vi "Power Values (Single Line).vi"(0 "phase voltage spectra":T2(array[cluster]), 5 "current spectra":T2(array[cluster]), 9 "system info in":refnum<class "EP System Info.lvclass">, 11 "error in (no error)":errorcluster) -> (4 "power values":T4, 6 "total power values":T3, 10 "system info out":refnum<class "EP System Info.lvclass">, 15 "error out":errorcluster)   [LabVIEW 2013, in "NI_EP_Power Quality.lvlib"]
doc: "Calculates the power values from the voltage and current spectra."
uses:
  <vilib>/addons/Electrical Power/PQ/NI_EP_Power Quality.lvlib
  <vilib>/addons/Electrical Power/PQ/Common/Classes/System Info/EP System Info.lvclass
  <vilib>/addons/Electrical Power/PQ/Common/Controls/ep_AI Data Channel.ctl
  <vilib>/addons/Electrical Power/Basic/NI_EP_Basic.lvlib
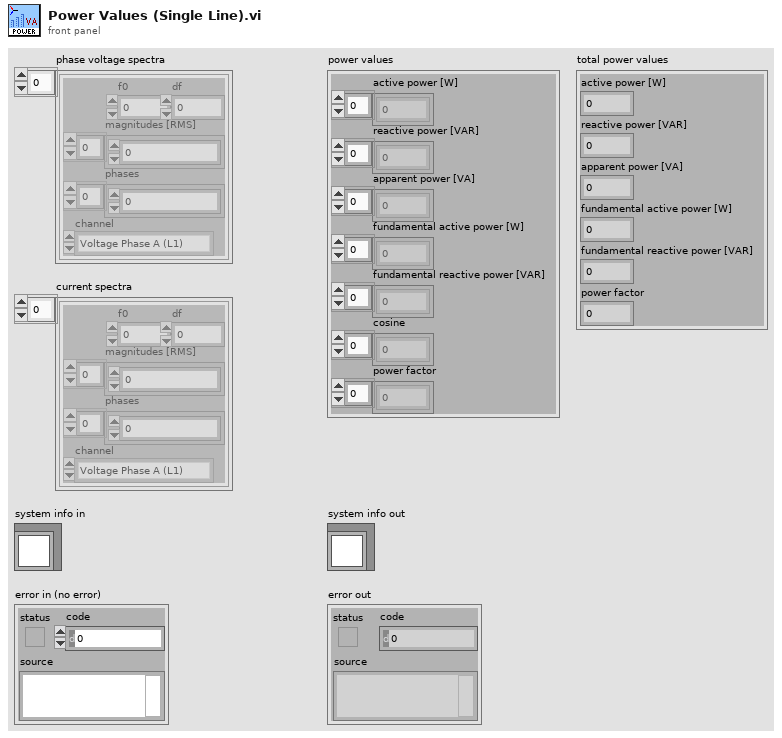
[diagram p1: front panel]
types:
  T1 = typedef "NI_EP_Power Quality.lvlib/ep_AI Data Channel.ctl" = enum16{"Voltage Phase A (L1)", "Voltage Phase B (L2)", "Voltage Phase C (L3)", "Voltage Phase N (Neutral)", "Current Phase A (L1)", "Current Phase B (L2)", "Current Phase C (L3)", "Current Phase N (Neutral)"}
  T2 = cluster{"f0":dbl, "df":dbl, "magnitudes [RMS]":dbl[], "phases":dbl[], "channel":T1}[]
  T3 = cluster{"active power [W]":dbl, "reactive power [VAR]":dbl, "apparent power [VA]":dbl, "fundamental active power [W]":dbl, "fundamental reactive power [VAR]":dbl, "power factor":dbl}
  T4 = cluster{"active power [W]":dbl[], "reactive power [VAR]":dbl[], "apparent power [VA]":dbl[], "fundamental active power [W]":dbl[], "fundamental reactive power [VAR]":dbl[], "cosine":dbl[], "power factor":dbl[]}
  T5 = cluster{"active power P (W)":dbl, "reactive power Q (VAr)":dbl, "apparent power S (VA)":dbl, "fundamental active power P1 (W)":dbl, "fundamental reactive power Q1 (VAr)":dbl, "power factor PF":dbl}
  T6 = cluster{"active power P (W)":dbl[], "reactive power Q (VAr)":dbl[], "apparent power S (VA)":dbl[], "fundamental active power P1 (W)":dbl[], "fundamental reactive power Q1 (VAr)":dbl[], "cosine":dbl[], "power factor PF":dbl[]}
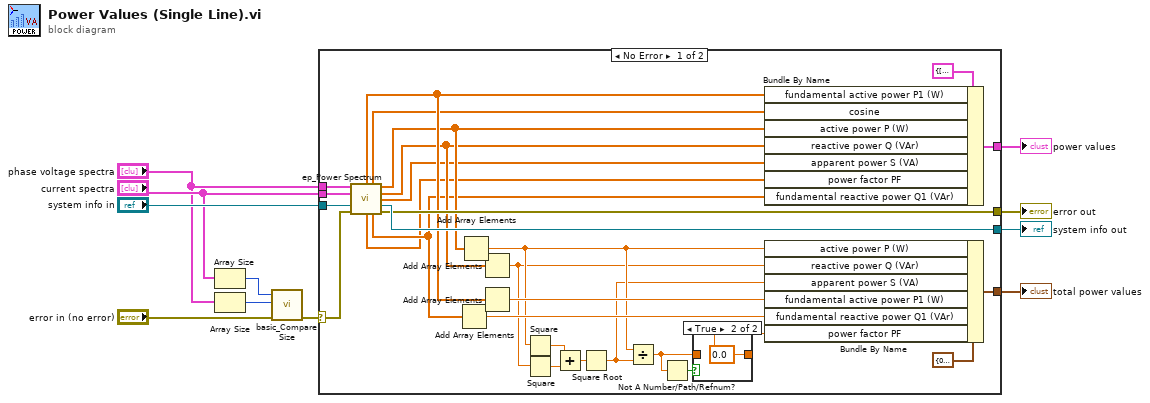
[diagram p0: block diagram]
diagram:
  n1 = Array Size(array="current spectra") -> (size(s)=w2:i32)
  n2 = Array Size(array="phase voltage spectra") -> (size(s)=w3:i32)
  n3 = call <vilib>:"basic_Compare Size.vi"("error in (no error)"="error in (no error)", "size B"=w3, "size A"=w2) -> ("error out"=w1:errorcluster)  [unwired: 8 in]
  n4 = case shown="No Error" w1 {
    selector: w1 -> [w18 w43]
    tunnel: [w39 _] -> w11
    tunnel: [w36 _] -> w10
    tunnel: "system info in" -> [w30 w42]
    tunnel: "current spectra" -> [w29 _]
    tunnel: "phase voltage spectra" -> [w28 _]
    tunnel: [w27 w42] -> w6
    tunnel: [w26 w43] -> w5
    frame No Error {
      n5 = call <vilib>:"ep_Power Spectrum.vi"("phase voltage spectra (5Hz step)"=w28, "current spectra (5Hz step)"=w29, "system info in"=w30, "error in (no error)"=w18) -> ("fundamental active power P1 (W)"=w25:dbl[], "cosine"=w24:dbl[], "active power P (W)"=w23:dbl[], "reactive power Q (VAr)"=w22:dbl[], "apparent power S (VA)"=w21:dbl[], "system info out"=w27:refnum<class "EP System Info.lvclass">, "power factor PF"=w19:dbl[], "fundamental reactive power Q1 (VAr)"=w20:dbl[], "error out"=w26:errorcluster)  [unwired: 3 in]
      n6 = Add Array Elements(numeric array=w20) -> (sum=w34:dbl)
      n7 = Add Array Elements(numeric array=w23) -> (sum=w17:dbl)
      n8 = Add Array Elements(numeric array=w22) -> (sum=w16:dbl)
      n9 = Add Array Elements(numeric array=w25) -> (sum=w35:dbl)
      n10 = Square(x=w17) -> (x^2=w15:dbl)
      n11 = Square(x=w16) -> (x^2=w14:dbl)
      n12 = Add(x=w15, y=w14) -> (x+y=w13:dbl)
      n13 = Square Root(x=w13) -> (sqrt(x)=w12:dbl)
      n14 = Divide(x=w17, y=w12) -> (x/y=w33:dbl)
      n15 = Not A Number/Path/Refnum?(number/path/refnum=w33) -> (NaN/Path/Refnum?=w32:bool)
      n16 = case shown="True" w32 {
        tunnel: w33 -> [w40 _]
        tunnel: [w40 0.0] -> w31
        frame False {
        }
        frame True {
        }
      }
      n17 = Bundle By Name(cluster=T6 {"active power P (W)"=[], "reactive power Q (VAr)"=[], "apparent power S (VA)"=[], "fundamental active power P1 (W)"=[], "fundamental reactive power Q1 (VAr)"=[], "cosine"=[], "power factor PF"=[]} ("power values"), "fundamental active power P1 (W)"=w25, "cosine"=w24, "active power P (W)"=w23, "reactive power Q (VAr)"=w22, "apparent power S (VA)"=w21, "power factor PF"=w19, "fundamental reactive power Q1 (VAr)"=w20) -> (w39:T6)
      n18 = Bundle By Name(cluster=T5 {"active power P (W)"=0.0, "reactive power Q (VAr)"=0.0, "apparent power S (VA)"=0.0, "fundamental active power P1 (W)"=0.0, "fundamental reactive power Q1 (VAr)"=0.0, "power factor PF"=0.0} ("total power"), "active power P (W)"=w17, "reactive power Q (VAr)"=w16, "apparent power S (VA)"=w12, "fundamental active power P1 (W)"=w35, "fundamental reactive power Q1 (VAr)"=w34, "power factor PF"=w31) -> (w36:T5)
    }
    frame Error {
    }
  }
  "error out" <- w5
  "power values" <- w11
  "system info out" <- w6
  "total power values" <- w10
